vi "SECoP_dataModifyScale.vi"(7 "Position":u32, 8 "error in (no error)":errorcluster, 9 "scale factor":dbl, 10 "SECoP_dataPtr":T1 {"ptr64" format="%.0x"; "ptr32" format="%.0x"}, 11 "DLL path (in)":T2) -> (0 "error out":errorcluster, 3 "DLL path (out)":T2)   [LabVIEW 2023, in "SECoP.lvlib"]
doc: "Call <b>\"SECoP_dataModifyScale.vi\"</b> to change the scale factor (SECoP_dataPtr).\n\n<b>DLL path</b> input and output of cluster from \"SECoP-Initialize.vi\"\n<b>SECoP_dataPtr</b> data to access\n<b>Position</b> points to a virtual flattened entry of the data type\n<b>scale factor</b> new scale factor of scaled value (non-zero)"
uses:
  SECoP.lvlib
  SECoP-libraries.ctl
  SECoP-data.ctl
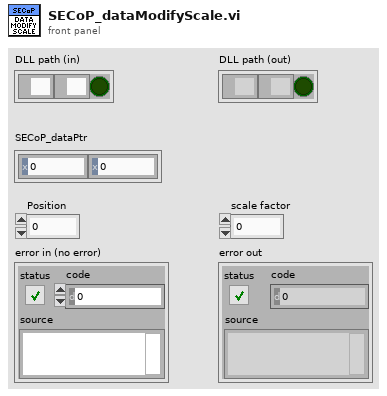
[diagram p1: front panel]
types:
  T1 = typedef "SECoP.lvlib/SECoP-data.ctl" = cluster{"ptr32":u32, "ptr64":u64}
  T2 = typedef "SECoP.lvlib/SECoP-libraries.ctl" = cluster{"serverDLL":path, "variantDLL":path, "cleanup_mode":bool}
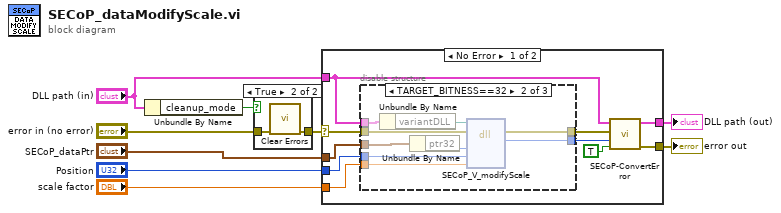
[diagram p0: block diagram]
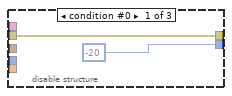
[diagram p3: hidden frame]
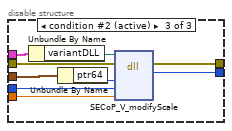
[diagram p4: hidden frame]
diagram:
  n1 = Unbundle By Name("DLL path (in)") -> ("cleanup_mode"=w6:bool)
  n2 = case shown="True" w6 {
    tunnel: "error in (no error)" -> [w10 w12]
    tunnel: [w10 w11] -> w4
    frame False {
    }
    frame True {
      n3 = call <vilib>:"Clear Errors.vi"("error in (no error)"=w12) -> ("error out"=w11:errorcluster)  [unwired: 5 in, 1 out]
    }
  }
  n4 = case shown="No Error" w4 {
    selector: w4 -> [w20 w43]
    tunnel: "DLL path (in)" -> [w13 w44]
    tunnel: [w21 w44] -> w8
    tunnel: [w22 w43] -> w7
    tunnel: "Position" -> [w16 _]
    tunnel: "SECoP_dataPtr" -> [w15 _]
    tunnel: "scale factor" -> [w14 _]
    frame No Error {
      n5 = disable-structure shown="TARGET_BITNESS==32" {
        disable-tunnel: w20 -> [w23 w33 w42]
        disable-tunnel: w13 -> [_ w26 w41]
        disable-tunnel: [w23 w32 w40] -> w19
        disable-tunnel: [-20 w31 w39] -> w18
        disable-tunnel: w16 -> [_ w30 w38]
        disable-tunnel: w15 -> [_ w28 w36]
        disable-tunnel: w14 -> [_ w27 w35]
        frame condition #0 {
        }
        frame condition #1 {
          n6 = Unbundle By Name(w26) -> ("variantDLL"=w25:path)
          n7 = Unbundle By Name(w28) -> ("ptr32"=w29:u32)
          n8 = dll-call lib="Z:/Praktische_Aufgaben/SECoP-LabVIEW2015/32bit/SECoP32.dll" fn="SECoP_V_modifyScale"(path in=w25, error in=w33, "pData"=w29, "uPosition"=w30, "dScale"=w27) -> (error out=w32:errorcluster, "return type"=w31:i32)  [unwired: 4 in, 1 out]
        }
        frame condition #2 (active) {
          n9 = Unbundle By Name(w41) -> ("variantDLL"=w34:path)
          n10 = Unbundle By Name(w36) -> ("ptr64"=w37:u64)
          n11 = dll-call lib="Z:/Praktische_Aufgaben/SECoP-LabVIEW2015/32bit/SECoP32.dll" fn="SECoP_V_modifyScale"(path in=w34, error in=w42, "pData"=w37, "uPosition"=w38, "dScale"=w35) -> (error out=w40:errorcluster, "return type"=w39:i32)  [unwired: 4 in, 1 out]
        }
      }
      n12 = call "SECoP-ConvertError.vi"("return is boolean"=TRUE, "return code"=w18, "error in (no error)"=w19, "DLL path (in)"=w13) -> ("error out"=w22:errorcluster, "DLL path (out)"=w21:T2)  [unwired: 6 in]
    }
    frame Error {
    }
  }
  "DLL path (out)" <- w8
  "error out" <- w7
